vi "ConfigComponent.vi"(10 "ActorAlias":string, 11 "ComponentActor":refnum<class "Actor.lvclass">) -> (3 "ComponentActorAlias":T1)   [LabVIEW 2020, in "jettl.lvlib"]
uses:
  jettl.lvlib
  Actor/Actor.lvclass
  ComponentActorAlias.ctl
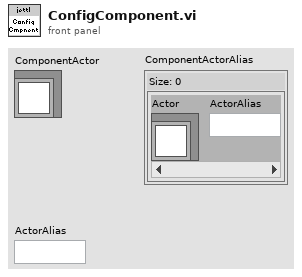
[diagram p1: front panel]
types:
  T1 = typedef "jettl.lvlib/ComponentActorAlias.ctl" = map{refnum<class "Actor.lvclass">, string}
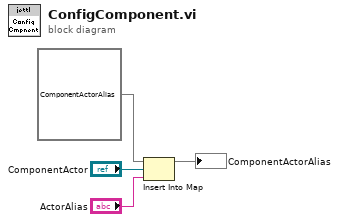
[diagram p0: block diagram]
diagram:
  n1 = Insert Into Map(map in=T1 {} ("ComponentActorAlias"), key="ComponentActor", value="ActorAlias") -> (map out=→"ComponentActorAlias":T1)  [unwired: 2 out]
